vi "FlatToRichmeasurement_StatusResponse.vi"(5 "OutputClusterType":T1, 11 "InputCluster":T2) -> (3 "OutputCluster":T1)   [LabVIEW 2021, in "Measurement_server.lvlib"]
uses:
  Measurement_server.lvlib
  measurement_StatusResponse_Flat.ctl
  measurement_StatusResponse.ctl
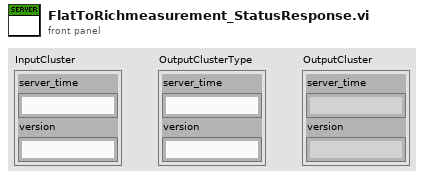
[diagram p1: front panel]
types:
  T1 = typedef "Measurement_server.lvlib/measurement_StatusResponse.ctl" = cluster{"server_time":string, "version":string}
  T2 = typedef "Measurement_server.lvlib/measurement_StatusResponse_Flat.ctl" = cluster{"server_time":string, "version":string}
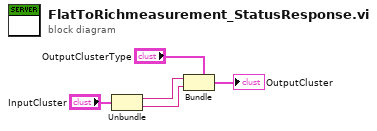
[diagram p0: block diagram]
diagram:
  n1 = Unbundle "Unbundle"("InputCluster") -> ("server_time"=w2:string, "version"=w1:string)
  n2 = Bundle "Bundle"(cluster="OutputClusterType", "server_time"=w2, "version"=w1) -> (→"OutputCluster":T1)
